vi "Add Error.vi"(8 "error in (no error)":errorcluster, 9 "String to Append":string, 10 "Error":T1, 11 "Insert Error":bool=TRUE) -> (0 "error out":errorcluster)   [LabVIEW 2021, in "Time_CIF_U.lvlib"]
uses:
  Time_CIF_U.lvlib
  Typedef/Errors.ctl
  Errors/Errors_CIF_U.lvlib
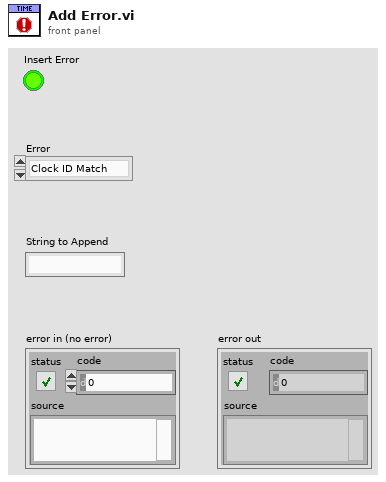
[diagram p1: front panel]
types:
  T1 = typedef "Time_CIF_U.lvlib/Errors.ctl" = enum16{"Clock ID Match", "Invalid Clock ID", "Long Sleep", "Linux Sleep"}
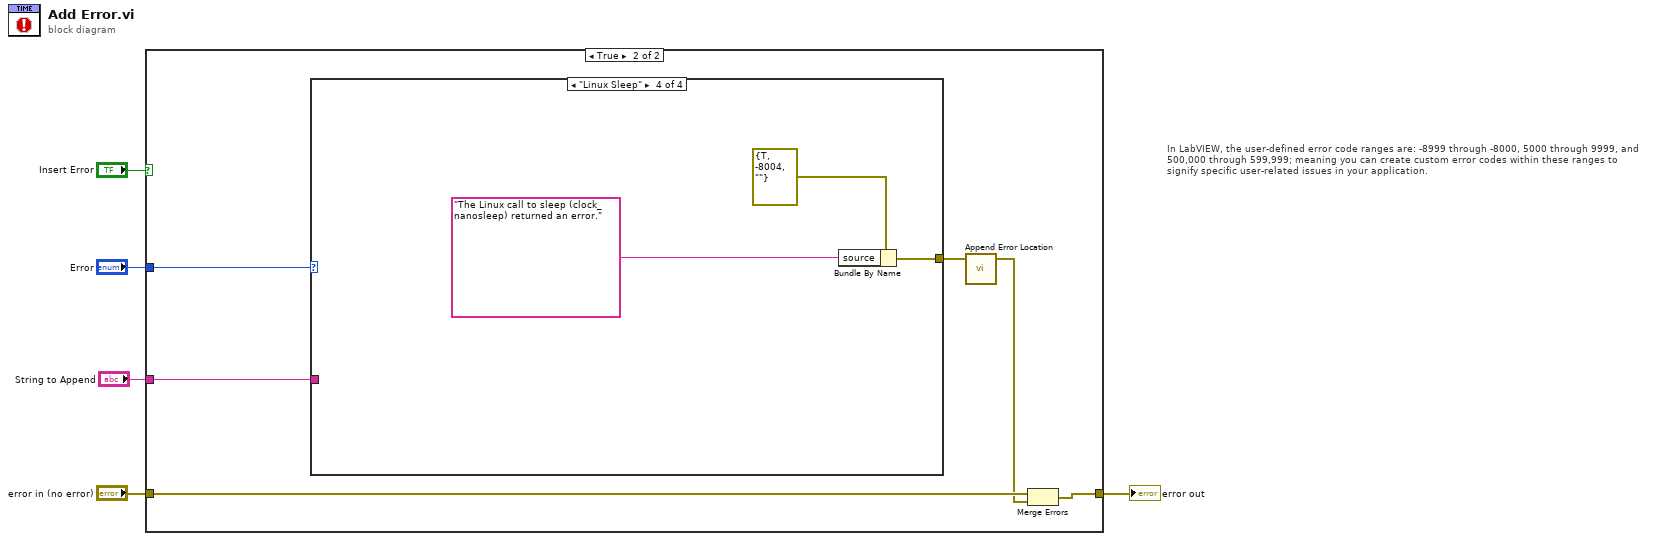
[diagram p0: block diagram]
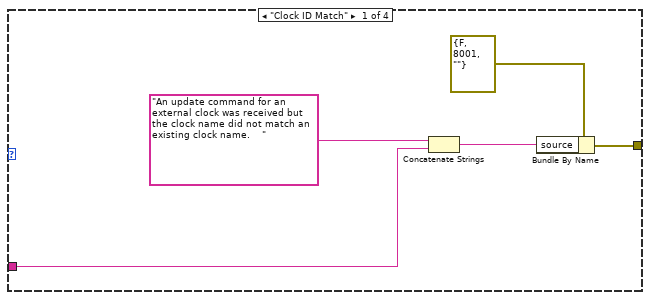
[diagram p3: hidden frame]
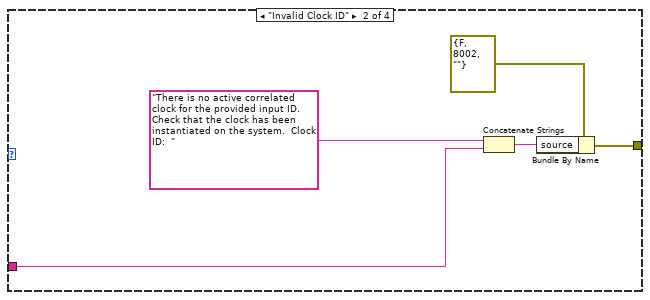
[diagram p4: hidden frame]
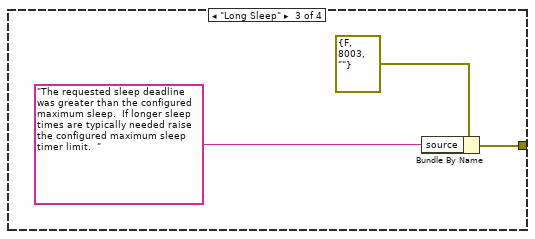
[diagram p5: hidden frame]
diagram:
  # "In LabVIEW, the user-defined error code ranges are: -8999 through -8000, 5000 through 9999, and 500,000 through 599,999; meaning you can create custom error codes within these ranges to signify specific user-related issues in your application."
  n1 = case shown="True" "Insert Error" {
    tunnel: [w6 w9] -> w4
    tunnel: "error in (no error)" -> [w6 w10]
    tunnel: "Error" -> [_ w12]
    tunnel: "String to Append" -> [_ w11]
    frame False {
    }
    frame True {
      n2 = case shown="\"Linux Sleep\"" w12 {
        tunnel: w11 -> [w13 w19 _ _]
        tunnel: [w16 w21 w24 w27] -> w8
        frame "Clock ID Match" {
          n3 = Concatenate Strings("An update command for an external clock was received but the clock name did not match an existing clock name.    " ("source"), w13) -> (w14:string)
          n4 = Bundle By Name(cluster=errorcluster {"status"=FALSE, "code"=8001, "source"=""} ("Invalid ID"), "source"=w14) -> (w16:errorcluster)
        }
        frame "Invalid Clock ID" {
          n5 = Concatenate Strings("There is no active correlated clock for the provided input ID.  Check that the clock has been instantiated on the system.  Clock ID:  " ("source"), w19) -> (w18:string)
          n6 = Bundle By Name(cluster=errorcluster {"status"=FALSE, "code"=8002, "source"=""} ("Invalid ID"), "source"=w18) -> (w21:errorcluster)
        }
        frame "Long Sleep" {
          n7 = Bundle By Name(cluster=errorcluster {"status"=FALSE, "code"=8003, "source"=""} ("Invalid ID"), "source"="The requested sleep deadline was greater than the configured maximum sleep.  If longer sleep times are typically needed raise the configured maximum sleep timer limit.  ") -> (w24:errorcluster)
        }
        frame "Linux Sleep" {
          n8 = Bundle By Name(cluster=errorcluster {"status"=TRUE, "code"=-8004, "source"=""} ("Invalid ID"), "source"="The Linux call to sleep (clock_nanosleep) returned an error.") -> (w27:errorcluster)
        }
      }
      n9 = call "Append Error Location.vi"("error in (no error)"=w8) -> ("error out"=w7:errorcluster)  [unwired: 4 in]
      n10 = Merge Errors(w10, w7) -> (w9:errorcluster)
    }
  }
  "error out" <- w4
